vi "Triangle process.vi"(0 "error in":errorcluster) -> ()   [LabVIEW 2012]
uses:
  Triangle global info.vi
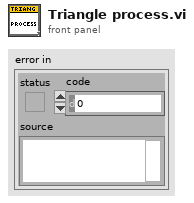
[diagram p1: front panel]
types:
  T1 = cluster{"Button 6":bool, "Button 7":bool, "Button 10":bool, "Button 11":bool, "Triangles values":dbl[]}
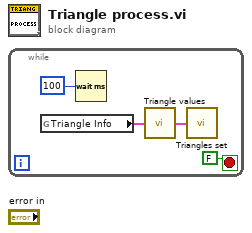
[diagram p0: block diagram]
diagram:
  n1 = while {
    stop <- FALSE stop-if-true
    n2 = global read "Triangle global info.vi" "Triangle Info"() -> (w3:T1)
    n3 = Wait (ms)(milliseconds to wait=u32 100) -> ()  [unwired: 1 out]
    n4 = call "Triangle values.vi"("Triangle Info"=w3) -> ("Triangle Info Out"=w4:T1)
    n5 = call "Triangles set.vi"("Triangle Info"=w4) -> ()
  }
